vi "Ticks To Inches.vi"(8 "error in":errorcluster, 11 "Ticks":dbl) -> (0 "error out":errorcluster, 3 "Inches":dbl)   [LabVIEW 2015]
panel:
  in  "Circumfrence (inches)":dbl=23.5
  in  "Ticks:Revolutions":dbl=1024.0
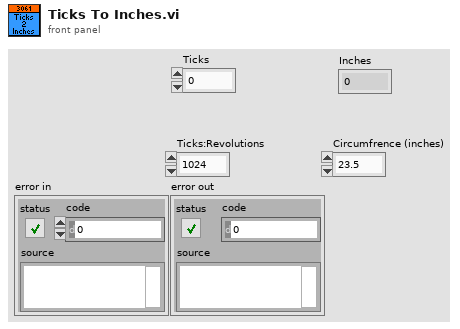
[diagram p1: front panel]
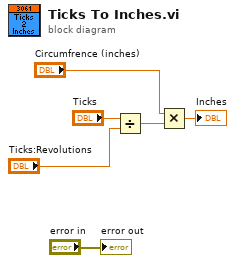
[diagram p0: block diagram]
diagram:
  n1 = Divide(x="Ticks", y="Ticks:Revolutions") -> (x/y=w4:dbl)
  n2 = Multiply(x="Circumfrence (inches)", y=w4) -> (x*y=→"Inches":dbl)
  "error out" <- "error in"
